vi "Module Init.vi"(8 "error in (no error)":errorcluster, 11 "SoftVar Module in":refnum<class "SoftVar Module.lvclass">) -> (0 "error out":errorcluster, 3 "SoftVar Module out":refnum<class "SoftVar Module.lvclass">)   [LabVIEW 2023, in "Volatus.lvlib" / "SoftVar Module.lvclass"]
uses:
  SoftVar Module.lvclass
  SoftVar Module.lvclass/SoftVar Module.ctl
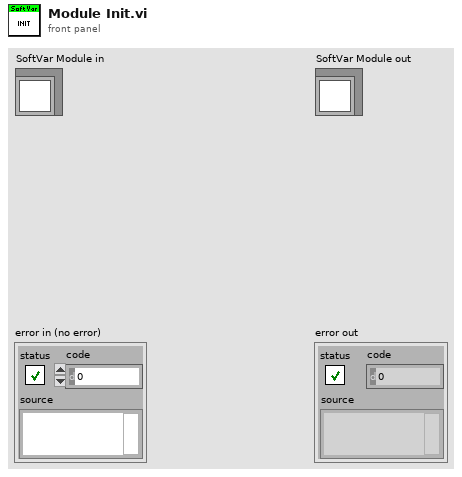
[diagram p1: front panel]
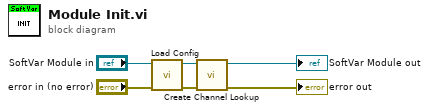
[diagram p0: block diagram]
diagram:
  n1 = call "Load Config.vi"("error in (no error)"="error in (no error)", "SoftVar Module in"="SoftVar Module in") -> ("error out"=w5:errorcluster, "SoftVar Module out"=w2:refnum<class "SoftVar Module.lvclass">)  [unwired: 8 in]
  n2 = call "Create Channel Lookup.vi"("error in (no error)"=w5, "SoftVar Module in"=w2) -> ("error out"=→"error out":errorcluster, "SoftVar Module out"=→"SoftVar Module out":refnum<class "SoftVar Module.lvclass">)  [unwired: 8 in]
